vi "Construct.vi"(8 "error in":errorcluster, 9 "logging configuration":T5, 10 "1553 Configuration":T1, 11 "device parameters":T7) -> (0 "error out":errorcluster, 3 "Ballard 1553 shared resources":refnum<class "Shared Resources.lvclass">)   [LabVIEW 2020, in "AIM MIL-STD-1553 Engine.lvlib" / "Implementation.lvlib" / "Shared Resources.lvclass"]
uses:
  Shared Resources.lvclass
  Shared/Initialization Method.ctl
  Shared/Device Parameters.ctl
  Shared/Data Word Format.ctl
  Custom Device/Logging Configuration.ctl
  Custom Device/Custom Device.lvlib
  Custom Device/Major Frame Configuration.ctl
  Custom Device/Minor Frame Configuration.ctl
  Custom Device/Message Configuration.ctl
  Custom Device/1553 Configuration.ctl
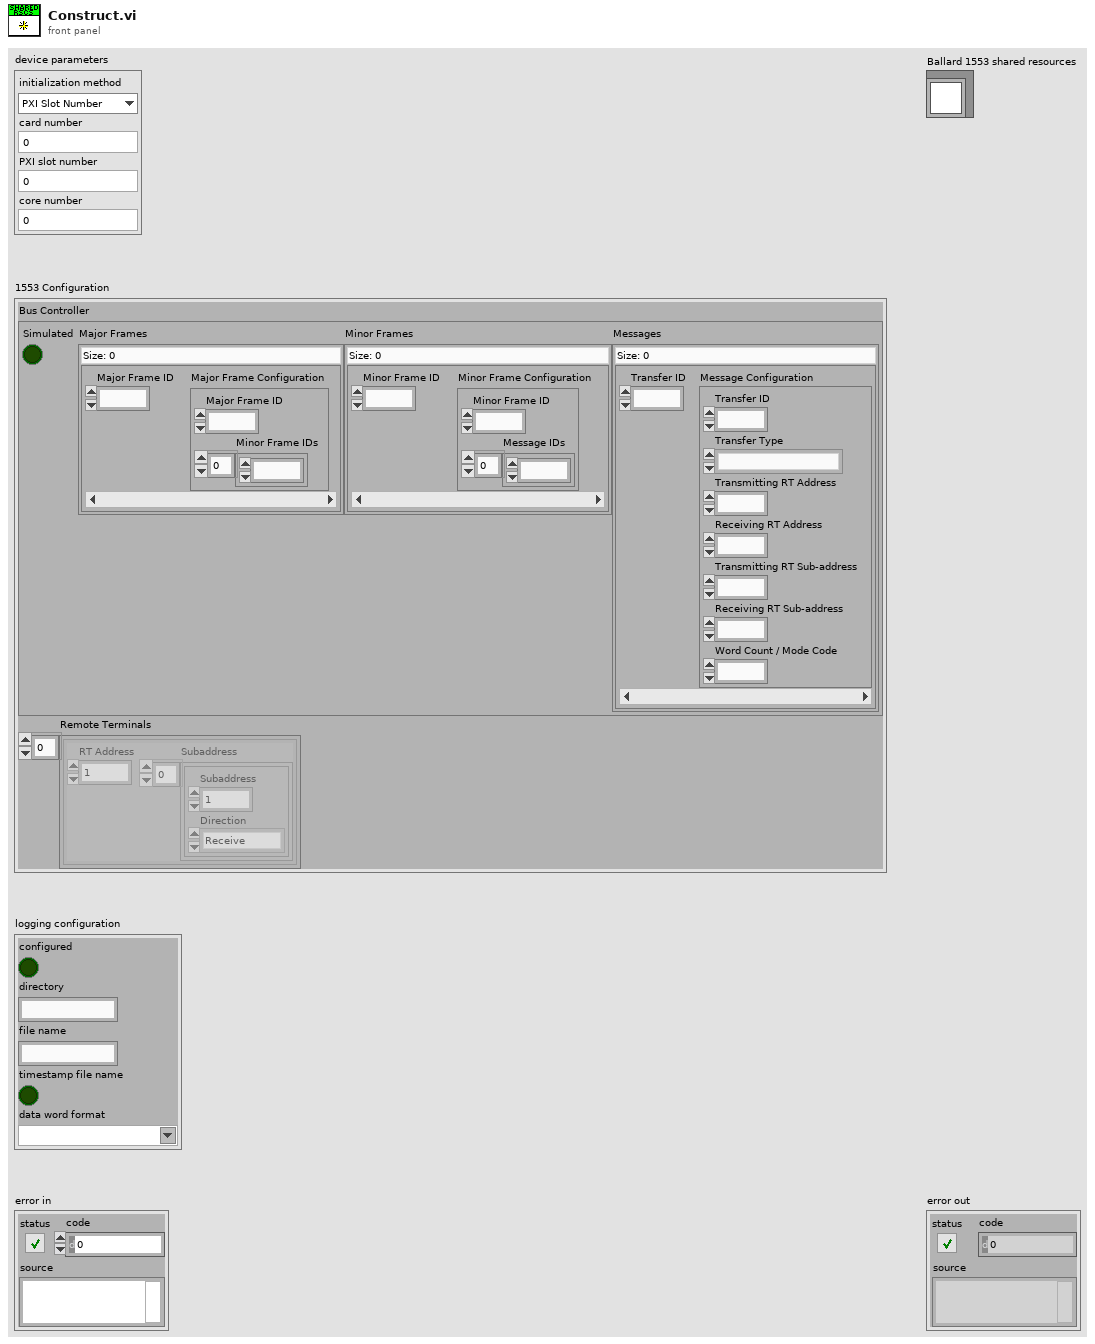
[diagram p1: front panel]
types:
  T1 = typedef "AIM MIL-STD-1553 Engine.lvlib/Custom Device.lvlib/1553 Configuration.ctl" = cluster{"Bus Controller":cluster{"Simulated":bool, "Major Frames":map{u16, T2}, "Minor Frames":map{u16, T3}, "Messages":map{u16, T4}}, "Remote Terminals":cluster{"RT Address":u8, "Subaddress":cluster{"Subaddress":u8, "Direction":enum16{"Receive", "Transmit"}}[]}[]}
  T2 = typedef "AIM MIL-STD-1553 Engine.lvlib/Custom Device.lvlib/Major Frame Configuration.ctl" = cluster{"Major Frame ID":u16, "Minor Frame IDs":u16[]}
  T3 = typedef "AIM MIL-STD-1553 Engine.lvlib/Custom Device.lvlib/Minor Frame Configuration.ctl" = cluster{"Minor Frame ID":u16, "Message IDs":u16[]}
  T4 = typedef "AIM MIL-STD-1553 Engine.lvlib/Custom Device.lvlib/Message Configuration.ctl" = cluster{"Transfer ID":u16, "Transfer Type":enum16{"BC to RT transfer", "RT to BC transfer", "RT to RT transfer"}, "Transmitting RT Address":u8, "Receiving RT Address":u8, "Transmitting RT Sub-address":u8, "Receiving RT Sub-address":u8, "Word Count / Mode Code":u8}
  T5 = typedef "AIM MIL-STD-1553 Engine.lvlib/Custom Device.lvlib/Logging Configuration.ctl" = cluster{"configured":bool, "directory":string, "file name":string, "timestamp file name":bool, "data word format":T6}
  T6 = typedef "Data Word Format.ctl" = string
  T7 = typedef "Device Parameters.ctl" = cluster{"initialization method":T8, "card number":i32, "PXI slot number":i32, "core number":i32}
  T8 = typedef "Initialization Method.ctl" = enum16{"PXI Slot Number", "Card Number"}
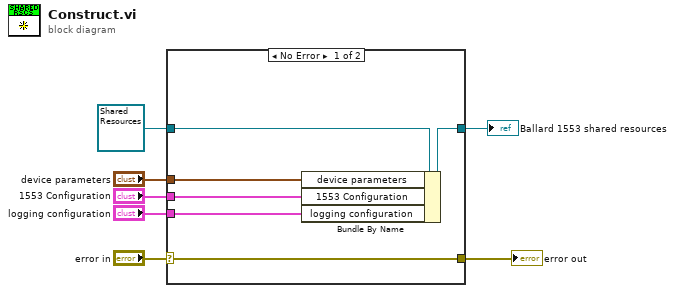
[diagram p0: block diagram]
diagram:
  n1 = case shown="No Error" "error in" {
    selector: "error in" -> [w11 w14]
    tunnel: refnum<class "Shared Resources.lvclass"> refnum ("Communication Bus Template Interfaces:Implementation.lvlib:Shared Resources.lvclass") -> [w13 w15]
    tunnel: [w12 w15] -> w6
    tunnel: [w11 w14] -> w4
    tunnel: "device parameters" -> [w10 _]
    tunnel: "logging configuration" -> [w9 _]
    tunnel: "1553 Configuration" -> [w8 _]
    frame No Error {
      n2 = Bundle By Name(cluster=w13, "device parameters"=w10, "1553 Configuration"=w8, "logging configuration"=w9) -> (w12:refnum<class "Shared Resources.lvclass">)
    }
    frame Error {
    }
  }
  "error out" <- w4
  "Ballard 1553 shared resources" <- w6
